vi "display_michelle_PKT_visjitter_stopadded_RandCont_PsuedoCO_TSLogFC1.vi"() -> ()   [LabVIEW 2019]
uses:
  <vilib>/Analysis/Matrix/Datatypes/RealMatrix.ctl
  <vilib>/Utility/file.llb/Write Delimited Spreadsheet (DBL).vi
  <vilib>/Analysis/Matrix/NI_Matrix.lvlib
panel:
  out "savecomplete":bool
  out "lambda":dbl
  out "maxITI":dbl
  out "minITI":dbl
  out "goEXP":dbl
  out "meanITI":dbl
  out "Lag1":dbl
  out "TSLog":dbl[][](array[numeric])
  out "TSLog2":dbl[][](array[numeric])
  out "Initialtime":dbl
  out "Time Stamp":timestamp format="%<%H:%M:%S%4u>T"
  out "TSLog1":dbl[][](array[numeric])
  out "ArrayTemp3":T1
  out "StimID2":dbl
  out "Contrast":dbl
  out "TimeOutCounter":i32
  out "ElapsedTime_M":dbl
  out "Base_Contrast":dbl
  out "CurrentTrial":u32=1
  out "Jitter":dbl
  out "BaseITI":dbl
  out "VisStimDuration":dbl
  in  "Stop":bool
  out "Num trials":u32=204
  out "ISI Time":dbl
  out "Stim TS":dbl
  out "Output":dbl[][](array[numeric])
  out "Output frame":T1
  out "Array temp1":T1
  out "Elapsed Time":dbl
  out "Display":bool=TRUE
  out "Trial":u32=1
  out "reward":dbl[](array[numeric])
  out "stim_id":dbl[](array[numeric])
  out "stim_loaded":dbl
  out "Timings":dbl[](array[numeric])
  out "Stimuli Loaded?":bool
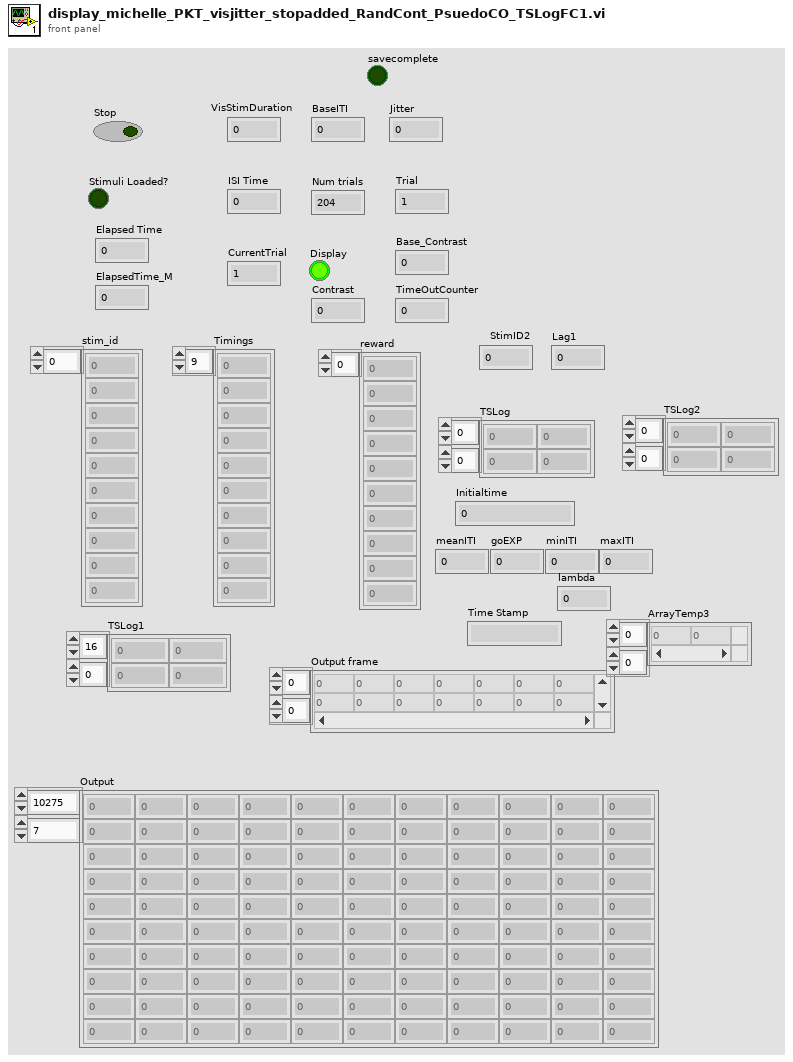
[diagram p1: front panel]
types:
  T1 = typedef "NI_Matrix.lvlib/RealMatrix.ctl" = dbl[][]
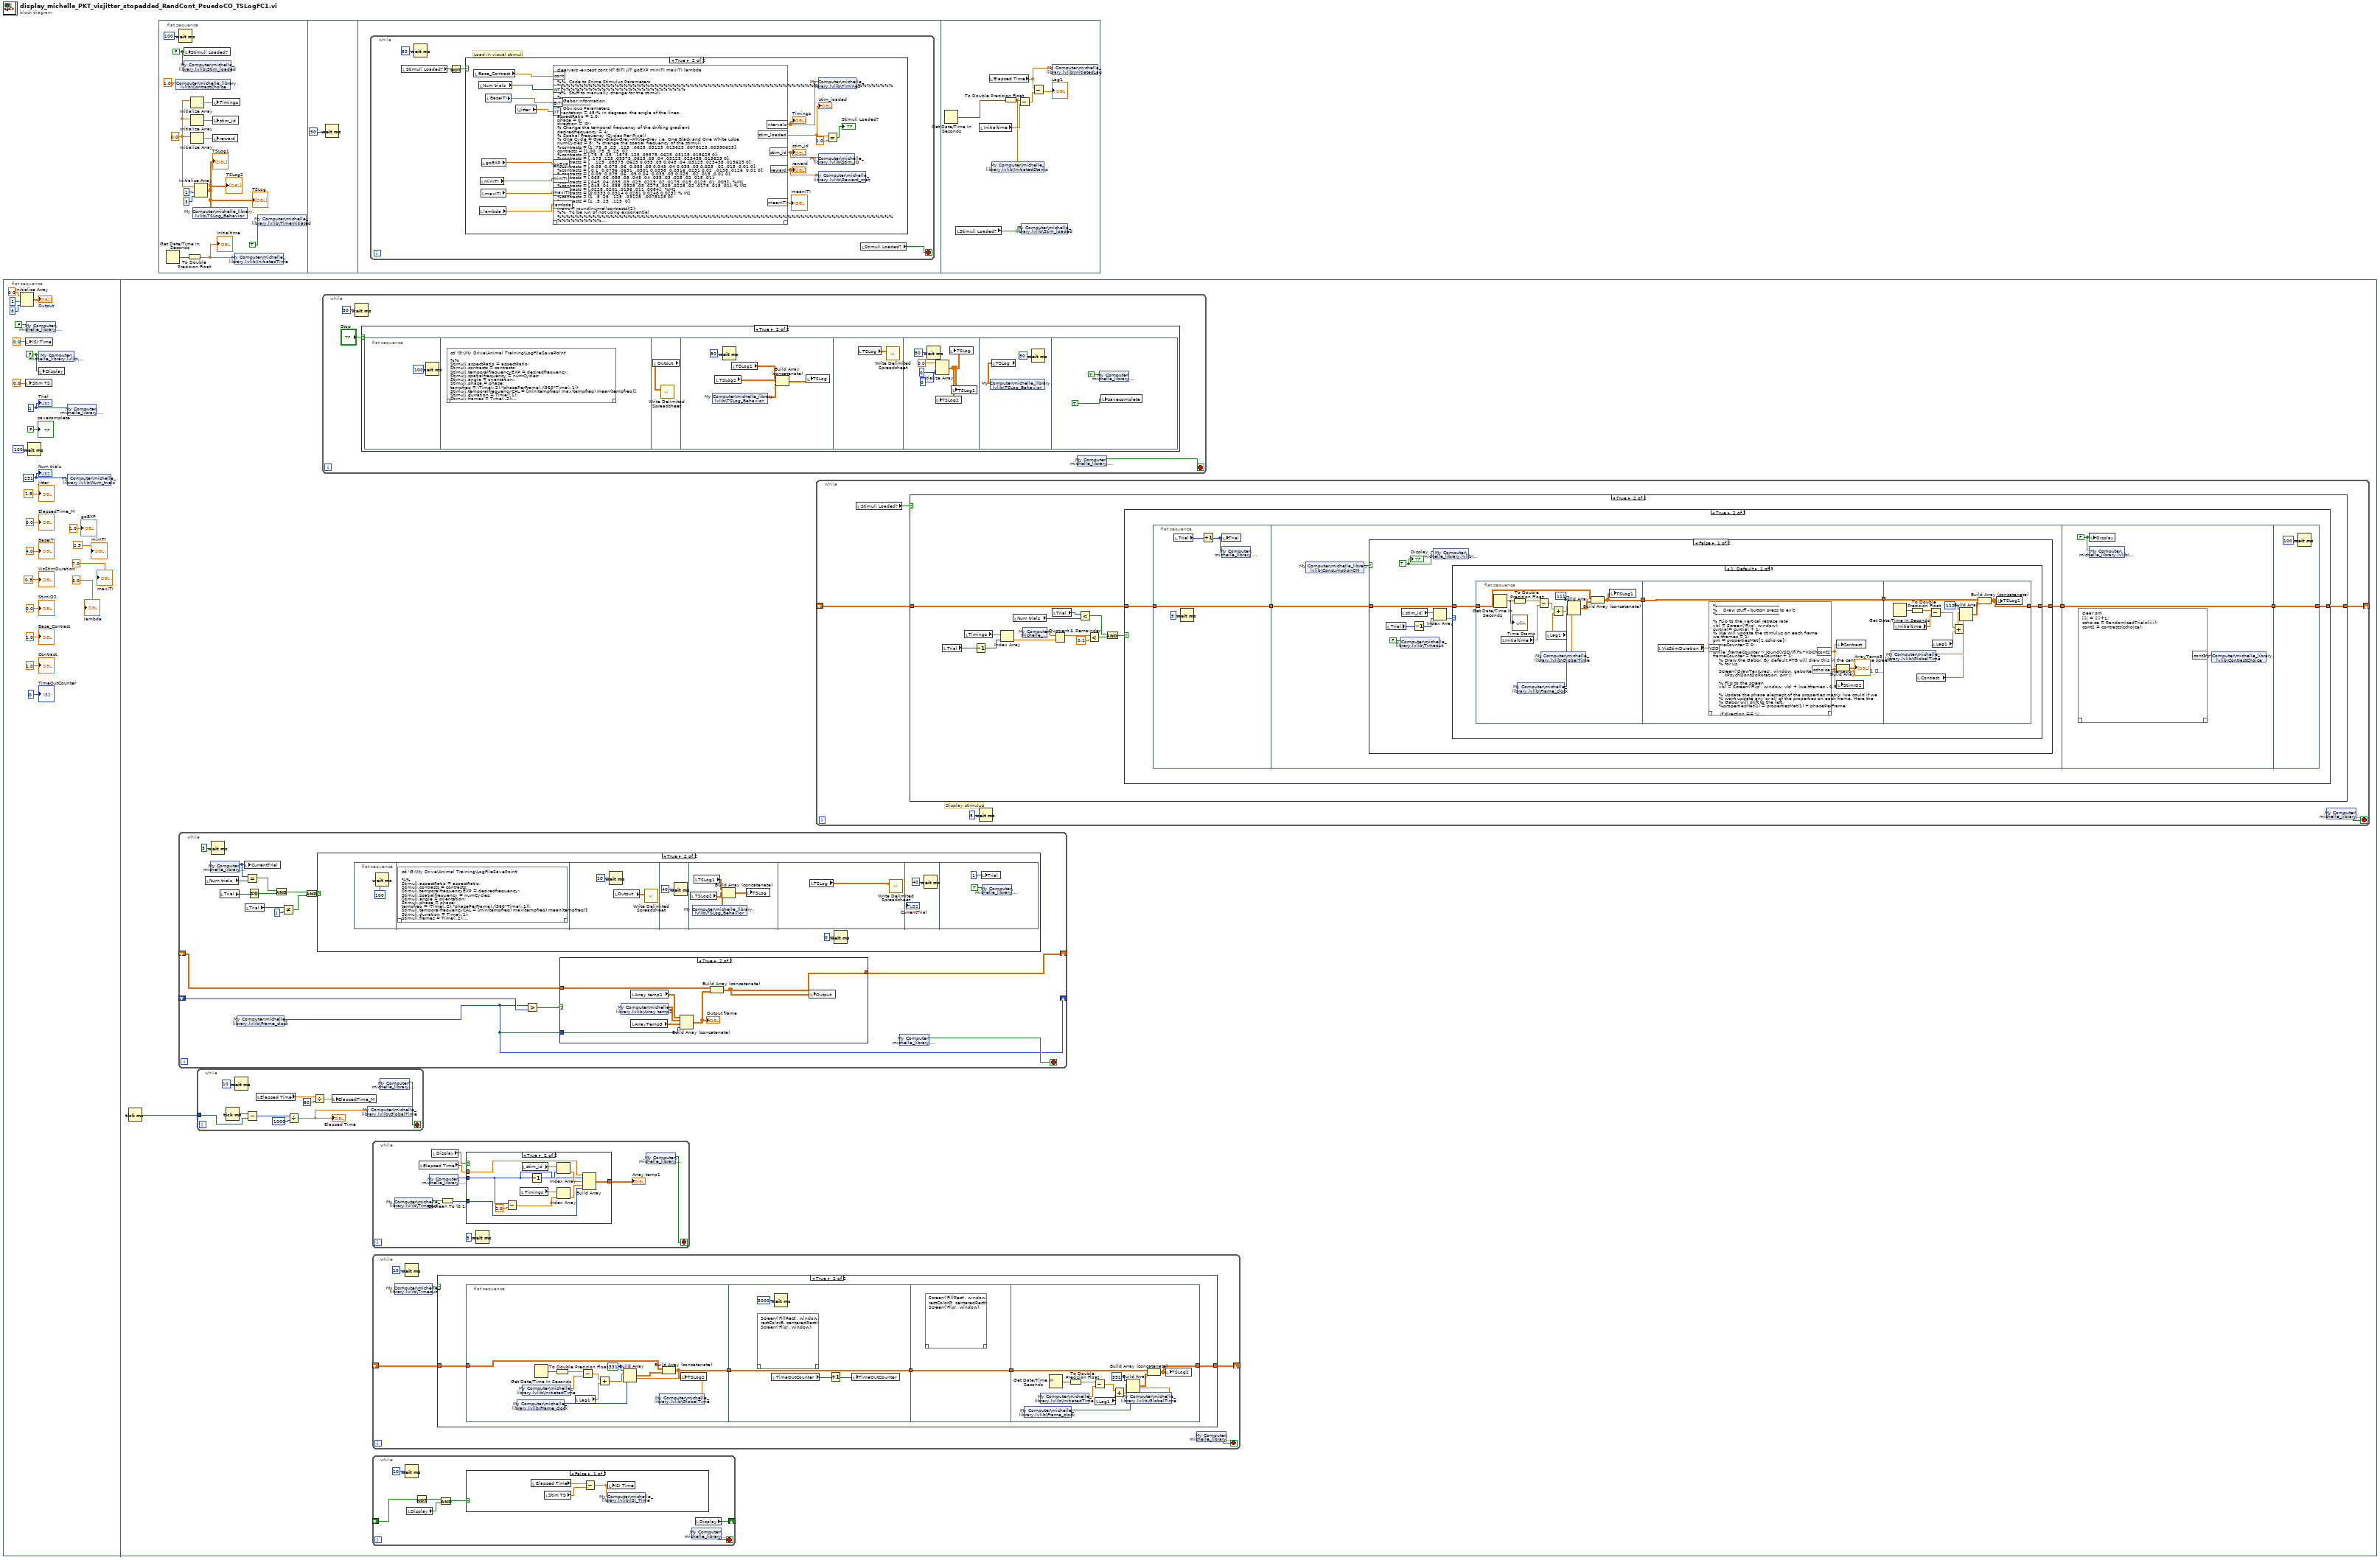
[diagram p0: block diagram]
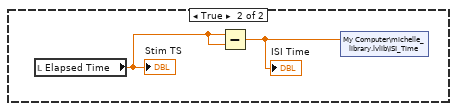
[diagram p5: hidden frame]
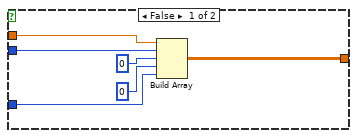
[diagram p6: hidden frame]
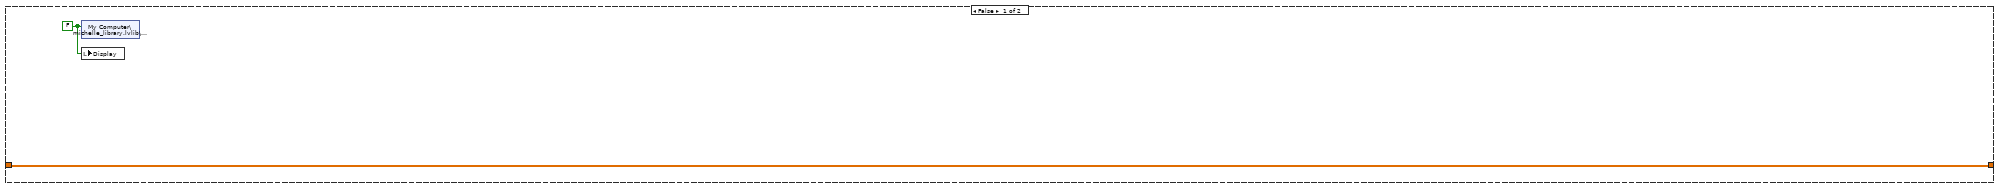
[diagram p10: hidden frame]
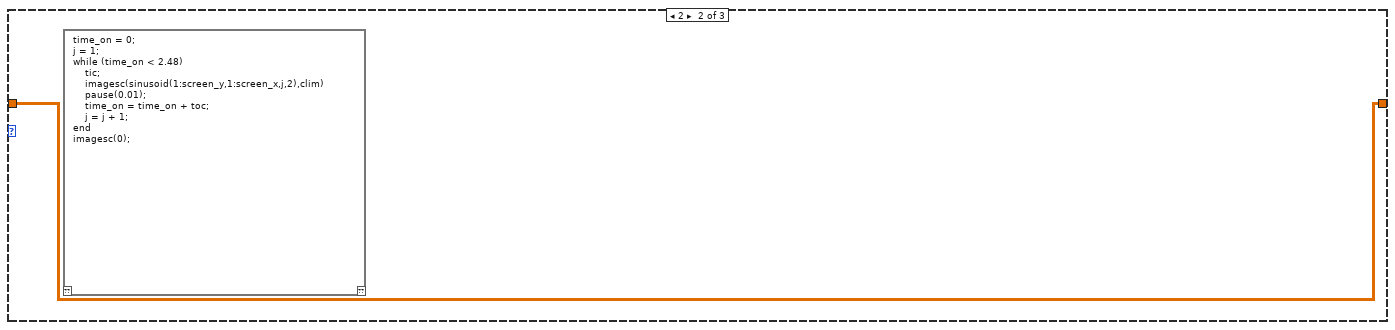
[diagram p11: hidden frame]
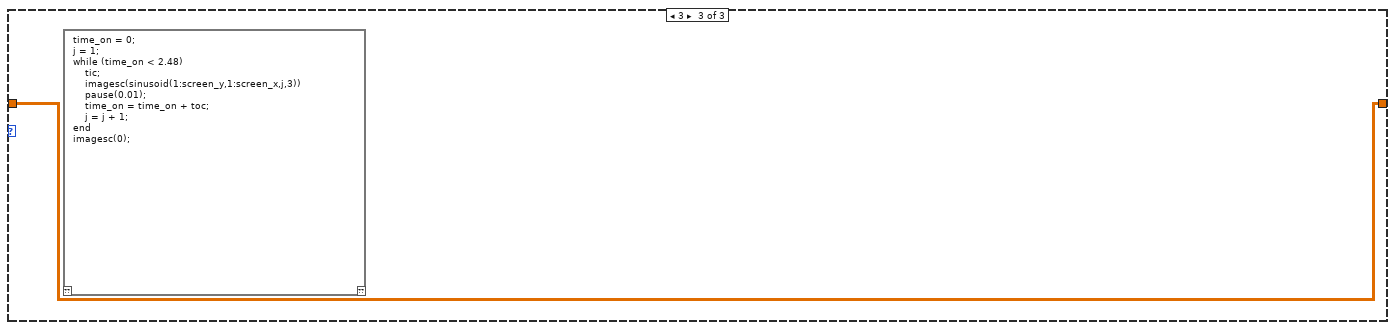
[diagram p12: hidden frame]
diagram:
  n1 = flat-sequence {
    frame #0 {
      w16 = u32 251
      w22 = FALSE ("Display")
      w24 = u32 1 ("Trial")
      n2 = Initialize Array(0.0 ("element"), 1 ("dimension size"), 8 ("dimension size")) -> (→"Output":dbl[][])
      n3 = local write "ISI Time"(0.0 ("ISI Time")) -> ()
      n4 = local write "Stim TS"(0.0 ("Stim TS")) -> ()
      n5 = shared-variable "My Computer\\michelle_library.lvlib\\Stop"(FALSE ("Stop")) -> ()  [unwired: 1 in, 1 out]
      n6 = Wait (ms)(milliseconds to wait=u32 100) -> ()  [unwired: 1 out]
      n7 = shared-variable "My Computer\\michelle_library.lvlib\\Display"(w22) -> ()  [unwired: 1 in, 1 out]
      n8 = local write "Display"(w22) -> ()
      n9 = shared-variable "My Computer\\michelle_library.lvlib\\Trial"(w24) -> ()  [unwired: 1 in, 1 out]
      n10 = shared-variable "My Computer\\michelle_library.lvlib\\Num_trials"(w16) -> ()  [unwired: 1 in, 1 out]
      "Trial" <- w24
      "Num trials" <- w16
      "VisStimDuration" <- 0.5
      "BaseITI" <- 4.0
      "Jitter" <- 1.5
      "Base_Contrast" <- 1.0
      "ElapsedTime_M" <- 0.0
      "TimeOutCounter" <- 0
      "Contrast" <- 1.0
      "StimID2" <- 0.0
      "goEXP" <- 1.0
      "minITI" <- 2.5
      "maxITI" <- 7.0
      "lambda" <- 6.0
      "savecomplete" <- FALSE
    }
    frame #1 {
      n11 = Tick Count (ms)() -> (millisecond timer value=w25:u32)
      n12 = while {
        shift-right: [w136] -> _
        shift-left: _ -> [w137]
        shift-right: [w133] -> _
        shift-left: _ -> [w135]
        stop <- w149 stop-if-true
        n13 = local read "Num trials"() -> (w147:u32)
        n14 = shared-variable "My Computer\\michelle_library.lvlib\\Trial"() -> (w138:u32)  [unwired: 1 in, 1 out]
        n15 = Wait (ms)(milliseconds to wait=u32 3) -> ()  [unwired: 1 out]
        n16 = local read "Trial"() -> (w145:u32)
        n17 = shared-variable "My Computer\\michelle_library.lvlib\\Frame_clock"() -> (w133:u32)  [unwired: 1 in, 1 out]
        n18 = local write "CurrentTrial"(w138) -> ()
        n19 = local read "Trial"() -> (w144:u32)
        n20 = Equal?(x=w138, y=w147) -> (x = y?=w146:bool)
        n21 = Not Equal To 0?(x=w145) -> (x != 0?=w141:bool)
        n22 = And(x=w146, y=w141) -> (x .and. y?=w139:bool)
        n23 = Not Equal?(x=w144, y=1) -> (x != y?=w143:bool)
        n24 = And(x=w139, y=w143) -> (x .and. y?=w140:bool)
        n25 = case shown="True" w140 {
          frame False {
          }
          frame True {
            n26 = flat-sequence {
              frame #0 {
                n27 = Wait (ms)(milliseconds to wait=100) -> ()  [unwired: 1 out]
              }
              frame #1 {
                n28 = script code="cd 'G:\\My Drive\\Animal Training\\LogFileSavePoint'\n\n%%\nStimuli.aspectRatio = aspectRatio;\nStimuli.contrasts = contrasts;\nStimuli.temporalfrequencyEXP = desiredfrequency;\nStimuli.spatialfrequency = numCycles;\nStimuli.angle = orientation;\nStimuli.phase = phase;\ntempfreq = (Time(:,2).*phasePerFrame)./(360*Time(:,1)); \nStimuli.temporalfrequencyCAL = [min(tempfreq) max(tempfreq) mean(tempfreq)];\nStimuli.durration = Time(:,1);\nStimuli.frames = Time(:,2);\nStimuli.contrast = Time(:,3);\nStimuli.intervals = intervals;\nif goEXP == 0\n     int.type = 'jitter';\n     int.baseITI = BITI;\n     int.jitter = JIT;\nelseif goEXP == 1\n     int.type = 'exponential';\n     int.minITI = minITI;\n     int.maxITI = maxITI;\n     int.lambda = lambda;\nend\nStimuli.IntervalData = int;\n\n\nWindow.Xpixels = screenXpixels;\nWindow.Ypixels = screenYpixels;\nWindow.Xcenter = xCenter;\nWindow.Ycenter = yCenter;\nWindow.ifi = ifi;\nWindow.screen = screenNumber;\n\n%%\n[logname] = generatelogname();\n\nsave(logname,'Stimuli','Window');\n\n%%"() -> ()  [unwired: 1 in, 1 out]
              }
              frame #2 {
                n29 = Wait (ms)(milliseconds to wait=u32 10) -> ()  [unwired: 1 out]
                n30 = local read "Output"() -> (w161:dbl[][])
                n31 = call-poly <vilib>:"Write Delimited Spreadsheet.vi"("2D data"=w161) -> ()  [unwired: 13 in, 2 out]
              }
              frame #3 {
                n32 = Wait (ms)(milliseconds to wait=u32 40) -> ()  [unwired: 1 out]
              }
              frame #4 {
                n33 = local read "TSLog2"() -> (w166:dbl[][])
                n34 = shared-variable "My Computer\\michelle_library.lvlib\\TSLog_Behavior"() -> (w164:dbl[][])  [unwired: 1 in, 1 out]
                n35 = local read "TSLog1"() -> (w165:dbl[][])
                n36 = Build Array (concatenate) ("Build Matrix")(w165, w166, w164) -> (w163:T1)
                n37 = local write "TSLog"(w163) -> ()
              }
              frame #5 {
                n38 = local read "TSLog"() -> (w167:dbl[][])
                n39 = call-poly <vilib>:"Write Delimited Spreadsheet.vi"("2D data"=w167) -> ()  [unwired: 13 in, 2 out]
              }
              frame #6 {
                n40 = Wait (ms)(milliseconds to wait=u32 40) -> ()  [unwired: 1 out]
              }
              frame #7 {
                n41 = local write "Trial"(1) -> ()
                n42 = shared-variable "My Computer\\michelle_library.lvlib\\Stop"(TRUE) -> ()  [unwired: 1 in, 1 out]
              }
            }
            n43 = Wait (ms)(milliseconds to wait=0) -> ()  [unwired: 1 out]
          }
        }
        n44 = Greater?(x=w133, y=w135) -> (0:w134:bool)
        n45 = case shown="True" w134 {
          tunnel: w137 -> [w150 w153]
          tunnel: [w150 w152] -> w136
          tunnel: w133 -> [_ w151]
          frame False {
          }
          frame True {
            n46 = shared-variable "My Computer\\michelle_library.lvlib\\Array temp2"() -> (w155:dbl[][])  [unwired: 1 in, 1 out]
            n47 = local read "Array temp1"() -> (w154:T1)
            n48 = local read "ArrayTemp3"() -> (w157:T1)
            n49 = Build Array (concatenate)(w154, w155, w157, w151) -> (w156:T1)
            "Output frame" <- w156
            n50 = Build Array (concatenate) ("Build Matrix")(w153, w156) -> (w152:T1)
            n51 = local write "Output"(w152) -> ()
          }
        }
        n52 = shared-variable "My Computer\\michelle_library.lvlib\\Stop"() -> (w149:bool)  [unwired: 1 in, 1 out]
      }
      n53 = while {
        tunnel: w25 -> [w130]
        stop <- w127 stop-if-true
        n54 = Tick Count (ms)() -> (millisecond timer value=w131:u32)
        n55 = Wait (ms)(milliseconds to wait=u32 10) -> ()  [unwired: 1 out]
        n56 = Subtract(x=w131, y=w130) -> (x-y=w128:u32)
        n57 = local read "Elapsed Time"() -> (w125:dbl)
        n58 = Divide(x=w128, y=u32 1000) -> (x/y=w123:dbl)
        "Elapsed Time" <- w123
        n59 = Divide(x=w125, y=60) -> (x/y=w124:dbl)
        n60 = local write "ElapsedTime_M"(w124) -> ()
        n61 = shared-variable "My Computer\\michelle_library.lvlib\\GlobalTime"(w123) -> ()  [unwired: 1 in, 1 out]
        n62 = shared-variable "My Computer\\michelle_library.lvlib\\Stop"() -> (w127:bool)  [unwired: 1 in, 1 out]
      }
      n63 = while {
        stop <- w26 stop-if-true
        n64 = Wait (ms)(milliseconds to wait=50) -> ()  [unwired: 1 out]
        n65 = case shown="True" "Stop" {
          frame False {
          }
          frame True {
            n66 = flat-sequence {
              frame #0 {
                n67 = Wait (ms)(milliseconds to wait=100) -> ()  [unwired: 1 out]
              }
              frame #1 {
                n68 = script code="cd 'G:\\My Drive\\Animal Training\\LogFileSavePoint'\n\n%%\nStimuli.aspectRatio = aspectRatio;\nStimuli.contrasts = contrasts;\nStimuli.temporalfrequencyEXP = desiredfrequency;\nStimuli.spatialfrequency = numCycles;\nStimuli.angle = orientation;\nStimuli.phase = phase;\ntempfreq = (Time(:,2).*phasePerFrame)./(360*Time(:,1)); \nStimuli.temporalfrequencyCAL = [min(tempfreq) max(tempfreq) mean(tempfreq)];\nStimuli.durration = Time(:,1);\nStimuli.frames = Time(:,2);\nStimuli.contrast = Time(:,3);\nStimuli.intervals = intervals;\nif goEXP == 0\n     int.type = 'jitter';\n     int.baseITI = BITI;\n     int.jitter = JIT;\nelseif goEXP == 1\n     int.type = 'exponential';\n     int.minITI = minITI;\n     int.maxITI = maxITI;\n     int.lambda = lambda;\nend\nStimuli.IntervalData = int;\n\n\nWindow.Xpixels = screenXpixels;\nWindow.Ypixels = screenYpixels;\nWindow.Xcenter = xCenter;\nWindow.Ycenter = yCenter;\nWindow.ifi = ifi;\nWindow.screen = screenNumber;\n\n%%\n[logname] = generatelogname();\n\nsave(logname,'Stimuli','Window');\n\n%%"() -> ()  [unwired: 1 in, 1 out]
              }
              frame #2 {
                n69 = local read "Output"() -> (w30:dbl[][])
                n70 = call-poly <vilib>:"Write Delimited Spreadsheet.vi"("2D data"=w30) -> ()  [unwired: 13 in, 2 out]
              }
              frame #3 {
                n71 = shared-variable "My Computer\\michelle_library.lvlib\\TSLog_Behavior"() -> (w31:dbl[][])  [unwired: 1 in, 1 out]
                n72 = local read "TSLog2"() -> (w34:dbl[][])
                n73 = Wait (ms)(milliseconds to wait=50) -> ()  [unwired: 1 out]
                n74 = local read "TSLog1"() -> (w33:dbl[][])
                n75 = Build Array (concatenate) ("Build Matrix")(w33, w34, w31) -> (w32:T1)
                n76 = local write "TSLog"(w32) -> ()
              }
              frame #4 {
                n77 = local read "TSLog"() -> (w36:dbl[][])
                n78 = call-poly <vilib>:"Write Delimited Spreadsheet.vi"("2D data"=w36) -> ()  [unwired: 13 in, 2 out]
              }
              frame #5 {
                n79 = Wait (ms)(milliseconds to wait=50) -> ()  [unwired: 1 out]
                n80 = Initialize Array(0.0, 0, 0) -> (w38:dbl[][])
                n81 = local write "TSLog2"(w38) -> ()
                n82 = local write "TSLog"(w38) -> ()
                n83 = local write "TSLog1"(w38) -> ()
              }
              frame #6 {
                n84 = local read "TSLog"() -> (w43:dbl[][])
                n85 = shared-variable "My Computer\\michelle_library.lvlib\\TSLog_Behavior"(w43) -> ()  [unwired: 1 in, 1 out]
                n86 = Wait (ms)(milliseconds to wait=50) -> ()  [unwired: 1 out]
              }
              frame #7 {
                n87 = shared-variable "My Computer\\michelle_library.lvlib\\Stop"(TRUE) -> ()  [unwired: 1 in, 1 out]
                n88 = local write "savecomplete"(TRUE) -> ()
              }
            }
          }
        }
        n89 = shared-variable "My Computer\\michelle_library.lvlib\\Stop"() -> (w26:bool)  [unwired: 1 in, 1 out]
      }
      n90 = while {
        stop <- w100 stop-if-true
        n91 = shared-variable "My Computer\\michelle_library.lvlib\\Timeout"() -> (w98:bool)  [unwired: 1 in, 1 out]
        n92 = local read "Elapsed Time"() -> (w104:dbl)
        n93 = shared-variable "My Computer\\michelle_library.lvlib\\Trial"() -> (w102:u32)  [unwired: 1 in, 1 out]
        n94 = local read "Display"() -> (w101:bool)
        n95 = Boolean To (0,1)(Boolean=w98) -> (0, 1=w99:i16)
        n96 = case shown="True" w101 {
          tunnel: w102 -> [w110 w113]
          tunnel: w104 -> [w111 w120]
          tunnel: [w109 w121] -> w103
          tunnel: w99 -> [w106 w115]
          frame False {
            n97 = Build Array(w111, w110, u32 0 ("milliseconds to wait"), 0, w106) -> (w109:T1)
          }
          frame True {
            n98 = Subtract(x=w113, y=2.0) -> (x-y=w112:dbl)
            n99 = local read "Timings"() -> (w118:dbl[])
            n100 = local read "stim_id"() -> (w122:dbl[])
            n101 = Decrement(x=w113) -> (x-1=w117:u32)
            n102 = Index Array(array=w122, index=w117) -> (element=w119:dbl)
            n103 = Index Array(array=w118, index=w112) -> (element=w116:dbl)
            n104 = Build Array(w120, w113, w119, w116, w115) -> (w121:T1)
          }
        }
        "Array temp1" <- w103
        n105 = Wait (ms)(milliseconds to wait=u32 5) -> ()  [unwired: 1 out]
        n106 = shared-variable "My Computer\\michelle_library.lvlib\\Stop"() -> (w100:bool)  [unwired: 1 in, 1 out]
      }
      n107 = while {
        shift-right: [w46] -> _
        shift-left: _ -> [w47]
        stop <- w50 stop-if-true
        n108 = shared-variable "My Computer\\michelle_library.lvlib\\Timeout"() -> (w48:bool)  [unwired: 1 in, 1 out]
        n109 = Wait (ms)(milliseconds to wait=u32 10) -> ()  [unwired: 1 out]
        n110 = case shown="True" w48 {
          tunnel: w47 -> [w51 w56]
          tunnel: [w51 w55] -> w46
          frame False {
          }
          frame True {
            n111 = flat-sequence {
              tunnel: w56 -> [w63]
              tunnel: [w62] -> w53
              tunnel: [w69] -> w54
              tunnel: w53 -> [w69]
              tunnel: w54 -> [w73]
              tunnel: [w73] -> w52
              tunnel: [w79] -> w55
              tunnel: w52 -> [w80]
              frame #0 {
                n112 = shared-variable "My Computer\\michelle_library.lvlib\\Frame_clock"() -> (w57:u32)  [unwired: 1 in, 1 out]
                n113 = shared-variable "My Computer\\michelle_library.lvlib\\InitiatedTime"() -> (w66:dbl)  [unwired: 1 in, 1 out]
                n114 = Get Date/Time In Seconds() -> (seconds since 1Jan1904=w68:timestamp)
                n115 = To Double Precision Float(number=w68) -> (double precision float=w67:dbl)
                n116 = local read "Lag1"() -> (w59:dbl)
                n117 = Subtract(x=w67, y=w66) -> (x-y=w60:dbl)
                n118 = Add(x=w60, y=w59) -> (x+y=w61:dbl)
                n119 = shared-variable "My Computer\\michelle_library.lvlib\\GlobalTime"() -> (w58:dbl)  [unwired: 1 in, 1 out]
                n120 = Build Array(331, w61, w58, w57) -> (w65:T1)
                n121 = Build Array (concatenate) ("Build Matrix")(w63, w65) -> (w62:T1)
                n122 = local write "TSLog2"(w62) -> ()
              }
              frame #1 {
                n123 = script code="Screen('FillRect', window, rectColorB, centeredRect);\nScreen('Flip', window);"() -> ()  [unwired: 1 in, 1 out]
                n124 = local read "TimeOutCounter"() -> (w71:i32)
                n125 = Wait (ms)(milliseconds to wait=u32 3000) -> ()  [unwired: 1 out]
                n126 = Increment(x=w71) -> (x+1=w70:i32)
                n127 = local write "TimeOutCounter"(w70) -> ()
              }
              frame #2 {
                n128 = script code="Screen('FillRect', window, rectColorG, centeredRect);\nScreen('Flip', window);"() -> ()  [unwired: 1 in, 1 out]
              }
              frame #3 {
                n129 = shared-variable "My Computer\\michelle_library.lvlib\\Frame_clock"() -> (w74:u32)  [unwired: 1 in, 1 out]
                n130 = shared-variable "My Computer\\michelle_library.lvlib\\InitiatedTime"() -> (w85:dbl)  [unwired: 1 in, 1 out]
                n131 = Get Date/Time In Seconds() -> (seconds since 1Jan1904=w83:timestamp)
                n132 = To Double Precision Float(number=w83) -> (double precision float=w84:dbl)
                n133 = Subtract(x=w84, y=w85) -> (x-y=w77:dbl)
                n134 = local read "Lag1"() -> (w76:dbl)
                n135 = Add(x=w77, y=w76) -> (x+y=w78:dbl)
                n136 = shared-variable "My Computer\\michelle_library.lvlib\\GlobalTime"() -> (w75:dbl)  [unwired: 1 in, 1 out]
                n137 = Build Array(332, w78, w75, w74) -> (w81:T1)
                n138 = Build Array (concatenate) ("Build Matrix")(w80, w81) -> (w79:T1)
                n139 = local write "TSLog2"(w79) -> ()
              }
            }
          }
        }
        n140 = shared-variable "My Computer\\michelle_library.lvlib\\Stop"() -> (w50:bool)  [unwired: 1 in, 1 out]
      }
      n141 = while {
        shift-right: [w90] -> _
        shift-left: _ -> [w89]
        stop <- w92 stop-if-true
        n142 = Wait (ms)(milliseconds to wait=u32 10) -> ()  [unwired: 1 out]
        n143 = local read "Display"() -> (w87:bool)
        n144 = Not(x=w89) -> (.not. x?=w88:bool)
        n145 = And(x=w88, y=w87) -> (x .and. y?=w86:bool)
        n146 = case shown="False" w86 {
          frame False {
            n147 = local read "Elapsed Time"() -> (w93:dbl)
            n148 = local read "Stim TS"() -> (w95:dbl)
            n149 = Subtract(x=w93, y=w95) -> (x-y=w94:dbl)
            n150 = local write "ISI Time"(w94) -> ()
            n151 = shared-variable "My Computer\\michelle_library.lvlib\\ISI_Time"(w94) -> ()  [unwired: 1 in, 1 out]
          }
          frame True {
            n152 = local read "Elapsed Time"() -> (w96:dbl)
            "Stim TS" <- w96
            n153 = Subtract(x=w96, y=w96) -> (x-y=w97:dbl)
            "ISI Time" <- w97
            n154 = shared-variable "My Computer\\michelle_library.lvlib\\ISI_Time"(w97) -> ()  [unwired: 1 in, 1 out]
          }
        }
        n155 = shared-variable "My Computer\\michelle_library.lvlib\\Stop"() -> (w92:bool)  [unwired: 1 in, 1 out]
        n156 = local read "Display"() -> (w90:bool)
      }
      n157 = while {
        shift-right: [w171] -> _
        shift-left: _ -> [w172]
        stop <- w174 stop-if-true
        # "Display stimulus"
        n158 = local read "Stimuli Loaded?"() -> (w173:bool)
        n159 = case shown="True" w173 {
          tunnel: w172 -> [w176 w178]
          tunnel: [w176 w177] -> w171
          frame False {
          }
          frame True {
            n160 = local read "Trial"() -> (w179:u32)
            n161 = local read "Timings"() -> (w188:dbl[])
            n162 = Decrement(x=w179) -> (x-1=w180:u32)
            n163 = Index Array(array=w188, index=w180) -> (element=w187:dbl)
            n164 = local read "Num trials"() -> (w183:u32)
            n165 = shared-variable "My Computer\\michelle_library.lvlib\\ISI"() -> (w182:dbl)  [unwired: 1 in, 1 out]
            n166 = local read "Trial"() -> (w186:u32)
            n167 = Quotient & Remainder(x=w182, y=w187) -> (x-y*floor(x/y)=w190:dbl)  [unwired: 1 out]
            n168 = Less?(x=w186, y=w183) -> (x < y?=w185:bool)
            n169 = Less?(x=w190, y=0.1) -> (x < y?=w184:bool)
            n170 = And(x=w185, y=w184) -> (x .and. y?=w181:bool)
            n171 = case shown="True" w181 {
              tunnel: w178 -> [w191 w196]
              tunnel: [w191 w195] -> w177
              frame False {
                w192 = FALSE ("Display")
                n172 = shared-variable "My Computer\\michelle_library.lvlib\\Display"(w192) -> ()  [unwired: 1 in, 1 out]
                n173 = local write "Display"(w192) -> ()
              }
              frame True {
                n174 = flat-sequence {
                  tunnel: [w198] -> w197
                  tunnel: w196 -> [w198]
                  tunnel: w197 -> [w203]
                  tunnel: [w202] -> w193
                  tunnel: [w249] -> w194
                  tunnel: w193 -> [w249]
                  tunnel: [w252] -> w195
                  tunnel: w194 -> [w252]
                  frame #0 {
                    n175 = local read "Trial"() -> (w201:u32)
                    n176 = Wait (ms)(milliseconds to wait=u32 5) -> ()  [unwired: 1 out]
                    n177 = Increment(x=w201) -> (x+1=w200:u32)
                    n178 = local write "Trial"(w200) -> ()
                    n179 = shared-variable "My Computer\\michelle_library.lvlib\\Trial"(w200) -> ()  [unwired: 1 in, 1 out]
                  }
                  frame #1 {
                    n180 = shared-variable "My Computer\\michelle_library.lvlib\\ConsumptionON"() -> (w204:bool)  [unwired: 1 in, 1 out]
                    n181 = case shown="False" w204 {
                      tunnel: w203 -> [w206 w248]
                      tunnel: [w205 w248] -> w202
                      frame False {
                        w207 = TRUE ("Boolean")
                        n182 = local read "Trial"() -> (w210:u32)
                        n183 = shared-variable "My Computer\\michelle_library.lvlib\\Timeout"(FALSE) -> ()  [unwired: 1 in, 1 out]
                        n184 = local read "stim_id"() -> (w212:dbl[])
                        n185 = Decrement(x=w210) -> (x-1=w209:u32)
                        n186 = shared-variable "My Computer\\michelle_library.lvlib\\Display"(w207) -> ()  [unwired: 1 in, 1 out]
                        n187 = Index Array(array=w212, index=w209) -> (element=w211:dbl)
                        n188 = case shown="1, Default" w211 {
                          tunnel: w206 -> [w216 w246 w247]
                          tunnel: [w215 w246 w247] -> w205
                          frame 1, Default {
                            n189 = flat-sequence {
                              tunnel: w216 -> [w227]
                              tunnel: [w226] -> w214
                              tunnel: w214 -> [w229]
                              tunnel: [w229] -> w213
                              tunnel: [w244] -> w215
                              tunnel: w213 -> [w243]
                              frame #0 {
                                n190 = Get Date/Time In Seconds() -> (seconds since 1Jan1904=w224:timestamp)
                                "Time Stamp" <- w224
                                n191 = local read "Initialtime"() -> (w222:dbl)
                                n192 = To Double Precision Float(number=w224) -> (double precision float=w223:dbl)
                                n193 = shared-variable "My Computer\\michelle_library.lvlib\\Frame_clock"() -> (w217:u32)  [unwired: 1 in, 1 out]
                                n194 = Subtract(x=w223, y=w222) -> (x-y=w220:dbl)
                                n195 = shared-variable "My Computer\\michelle_library.lvlib\\GlobalTime"() -> (w218:dbl)  [unwired: 1 in, 1 out]
                                n196 = local read "Lag1"() -> (w221:dbl)
                                n197 = Add(x=w220, y=w221) -> (x+y=w219:dbl)
                                n198 = Build Array(111, w219, w218, w217) -> (w225:T1)
                                n199 = Build Array (concatenate) ("Build Matrix")(w227, w225) -> (w226:T1)
                                n200 = local write "TSLog1"(w226) -> ()
                              }
                              frame #1 {
                                n201 = local read "VisStimDuration"() -> (w231:dbl)
                                n202 = script code="%------------------------------------------\n%    Draw stuff - button press to exit\n%------------------------------------------\n\n% FLip to the vertical retrace rate\nvbl = Screen('Flip', window);\ncurtrial= curtrial + 1;\n% We will update the stimulus on each frame\nwaitframes = 1;\npm = propertiesMat{1,cchoice};\nframeCounter = 0;\ntic\nwhile  frameCounter < round(VSD/ifi)%~KbCheck\nframeCounter = frameCounter + 1;\n    % Draw the Gabor. By default PTB will draw this in the center of the screen\n    % for us.\n   \n    Screen('DrawTextures', window, gabortex, [], [], orientation, [], [], [], [],...\n        kPsychDontDoRotation, pm');\n\n    % Flip to the screen\n    vbl = Screen('Flip', window, vbl + (waitframes - 0.5) * ifi);\n\n    % Update the phase element of the properties matrix (we could if we\n    % want update any or all of the properties on each frame. Here the\n    % Gabor will drift to the left.\n    %propertiesMat(1) = propertiesMat(1) + phasePerFrame;\n \n     if direction == 'L'\n          pm(1) = pm(1) + phasePerFrame;\n     elseif direction =='R'\n          pm(1) = pm(1) - phasePerFrame;\n     end\n\nend\nTime(curtrial,1) = toc;\nTime(curtrial,2) = frameCounter;\nTime(curtrial,3) = pm(4);\nvbl = Screen('Flip', window);"("VSD"=w231) -> ("cont2"=w233:dbl, "cchoice"=w232:dbl)  [unwired: 1 in, 1 out]
                                n203 = local write "Contrast"(w233) -> ()
                                n204 = Build Array(w233, w232) -> (→"ArrayTemp3":T1)
                                n205 = local write "StimID2"(w232) -> ()
                              }
                              frame #2 {
                                n206 = shared-variable "My Computer\\michelle_library.lvlib\\GlobalTime"() -> (w235:dbl)  [unwired: 1 in, 1 out]
                                n207 = Get Date/Time In Seconds() -> (seconds since 1Jan1904=w241:timestamp)
                                n208 = local read "Initialtime"() -> (w240:dbl)
                                n209 = To Double Precision Float(number=w241) -> (double precision float=w239:dbl)
                                n210 = local read "Contrast"() -> (w234:dbl)
                                n211 = Subtract(x=w239, y=w240) -> (x-y=w238:dbl)
                                n212 = local read "Lag1"() -> (w236:dbl)
                                n213 = Add(x=w238, y=w236) -> (x+y=w237:dbl)
                                n214 = Build Array(112, w237, w235, w234) -> (w245:T1)
                                n215 = Build Array (concatenate) ("Build Matrix")(w243, w245) -> (w244:T1)
                                n216 = local write "TSLog1"(w244) -> ()
                              }
                            }
                          }
                          frame 2 {
                            n217 = script code="time_on = 0;\nj = 1;\nwhile (time_on < 2.48)\n    tic;\n    imagesc(sinusoid(1:screen_y,1:screen_x,j,2),clim)\n    pause(0.01);\n    time_on = time_on + toc;\n    j = j + 1;\nend\nimagesc(0);"() -> ()  [unwired: 1 in, 1 out]
                          }
                          frame 3 {
                            n218 = script code="time_on = 0;\nj = 1;\nwhile (time_on < 2.48)\n    tic;\n    imagesc(sinusoid(1:screen_y,1:screen_x,j,3))\n    pause(0.01);\n    time_on = time_on + toc;\n    j = j + 1;\nend\nimagesc(0);"() -> ()  [unwired: 1 in, 1 out]
                          }
                        }
                        "Display" <- w207
                      }
                      frame True {
                      }
                    }
                  }
                  frame #2 {
                    w251 = FALSE ("Display")
                    n219 = script code="clear pm\niiii = iiii+1;\ncchoice = RandomizedTrials(iiii);\ncont2 = contrasts(cchoice);"() -> ("cont2"=w250:dbl)  [unwired: 1 in, 1 out]
                    n220 = local write "Display"(w251) -> ()
                    n221 = shared-variable "My Computer\\michelle_library.lvlib\\Display"(w251) -> ()  [unwired: 1 in, 1 out]
                    n222 = shared-variable "My Computer\\michelle_library.lvlib\\ContrastChoice"(w250) -> ()  [unwired: 1 in, 1 out]
                  }
                  frame #3 {
                    n223 = Wait (ms)(milliseconds to wait=u32 100) -> ()  [unwired: 1 out]
                  }
                }
              }
            }
          }
        }
        n224 = Wait (ms)(milliseconds to wait=u32 5) -> ()  [unwired: 1 out]
        n225 = shared-variable "My Computer\\michelle_library.lvlib\\Stop"() -> (w174:bool)  [unwired: 1 in, 1 out]
      }
    }
  }
  n226 = flat-sequence {
    frame #0 {
      w260 = 0.0 ("element")
      w262 = FALSE ("Stimuli Loaded?")
      n227 = Get Date/Time In Seconds() -> (seconds since 1Jan1904=w257:timestamp)
      n228 = shared-variable "My Computer\\michelle_library.lvlib\\ContrastChoice"(1.0) -> ()  [unwired: 1 in, 1 out]
      n229 = Wait (ms)(milliseconds to wait=u32 100) -> ()  [unwired: 1 out]
      n230 = local write "Stimuli Loaded?"(w262) -> ()
      n231 = shared-variable "My Computer\\michelle_library.lvlib\\Stim_loaded"(w262) -> ()  [unwired: 1 in, 1 out]
      n232 = To Double Precision Float(number=w257) -> (double precision float=w256:dbl)
      "Initialtime" <- w256
      n233 = Initialize Array(w260) -> (w265:dbl[])  [unwired: 1 in]
      n234 = Initialize Array(w260) -> (w264:dbl[])  [unwired: 1 in]
      n235 = Initialize Array(w260) -> (w263:dbl[])  [unwired: 1 in]
      n236 = Initialize Array(w260, 1, 3) -> (w254:dbl[][])
      "TSLog1" <- w254
      "TSLog2" <- w254
      "TSLog" <- w254
      n237 = shared-variable "My Computer\\michelle_library.lvlib\\TSLog_Behavior"(w254) -> ()  [unwired: 1 in, 1 out]
      n238 = local write "Timings"(w265) -> ()
      n239 = local write "stim_id"(w264) -> ()
      n240 = local write "reward"(w263) -> ()
      n241 = shared-variable "My Computer\\michelle_library.lvlib\\InitiatedTime"(w256) -> ()  [unwired: 1 in, 1 out]
      n242 = shared-variable "My Computer\\michelle_library.lvlib\\TimeInitiated"(TRUE) -> ()  [unwired: 1 in, 1 out]
    }
    frame #1 {
      n243 = Wait (ms)(milliseconds to wait=u32 50) -> ()  [unwired: 1 out]
    }
    frame #2 {
      n244 = while {
        stop <- w268 stop-if-true
        # "Load in visual stimuli"
        n245 = local read "Stimuli Loaded?"() -> (w270:bool)
        n246 = Wait (ms)(milliseconds to wait=u32 50) -> ()  [unwired: 1 out]
        n247 = Not(x=w270) -> (.not. x?=w269:bool)
        n248 = case shown="True" w269 {
          frame False {
          }
          frame True {
            n249 = local read "Base_Contrast"() -> (w278:dbl)
            n250 = local read "Num trials"() -> (w281:u32)
            n251 = local read "lambda"() -> (w272:dbl)
            n252 = local read "minITI"() -> (w274:dbl)
            n253 = local read "maxITI"() -> (w273:dbl)
            n254 = local read "goEXP"() -> (w275:dbl)
            n255 = local read "BaseITI"() -> (w280:dbl)
            n256 = local read "Jitter"() -> (w279:dbl)
            n257 = script code="clearvars -except cont NT BITI JIT goEXP minITI maxITI lambda\n\n\n%%  Code to Prime Stimulus Parameters\n%%%%%%%%%%%%%%%%%%%%%%%%%%%%%%%%%%%%%%%%%%%%%%%%%%%%%%%%%%%%%%%%%%%%%%%%%%%%%%%%%%%%%%%%%%%%%%%%%%%%%%%%%\n%%  Stuff to manually change for the stimuli\n%--------------------\n% Gabor information\n%--------------------\n% Obvious Parameters\norientation = 45;% in degrees, the angle of the lines.\naspectRatio = 1.0;\nphase = 0;\ndirection = 'R';\n% Change the temporal frequency of the drifting gradient\ndesiredfrequency = 4;\n% Spatial Frequency (Cycles Per Pixel)\n% One Cycle = Grey-Black-Grey-White-Grey i.e. One Black and One White Lobe\nnumCycles = 8;  % change the spatial frequency of the stimuli\n%contrasts = [1 .75 .5 .25  .125  .0625 .03125 .015625 .0078125 .00390625];\ncontrasts = [1.00 .75 .5 .25  0];\n%contrasts = [.75 .5 .25  .1875 .125 .09375 .0625 .03125 .015625 0];\n%contrasts = [ .175 .125 .09375 .0625 .05 .04 .03125 .023438 .015625 0];\n%contrasts = [   .125  .09375 .0625 0.055 .05 0.045 .04 .03125 .023438 .015625 0];\n%contrasts = [ 0.09  0.075 .06  0.055 .05 0.045 .04 0.035 .03 0.025  .02 .015  0.01 0];\n%contrasts = [ 0.1  0.0796 .0631  .0501 0.0398  0.0316 .0251 0.02  .0158 .0126  0.01 0];\n%contrasts = [ 0.09  0.075 .06  .05 0.04  0.035 .03 0.025  .02 .015  0.01 0];\n%contrasts = [.065 .06 .055 .05 .045 .04 .035 .03 .025 .02 .015 .01];\n%contrasts = [.045 .04 .035 .03 .025 .0225 .02 .0175 .015 .0125 .01 .005];  %M1\n%contrasts = [.045 .04 .035 .0325 .03 .0275 .025 .0225 .02 .0175 .015 .01]; % M2\n%contrasts = [.0228 .0201 .0156 .011 .0084];  %M1\n%contrasts = [0.0333 0.0314 0.0281 0.0248 0.023]; % M2\n%contrasts = [1  .5 .25  .125  .03125  .0078125 0];\n%contrasts = [1  .5 .25  .125  0];\ngo = 1;\nmaxc = round(numel(contrasts)/2);\n%%  To be run of not using exponential\n%%%%%%%%%%%%%%%%%%%%%%%%%%%%%%%%%%%%%%%%%%%%%%%%%%%%%%%%%%%%%%%%%%%%%%%%%%%%%%%%%%%%%%\n% This code will randomize the order of contrasts being presented\n[RandomizedTrials]=RandomizeTrials_Psuedo_function(contrasts,NT,'n');\n\n% This code will generate inter trial intervals with either random jitter\n% or based on an exponential distribution\nif goEXP < 1\n     jit = JIT;\n     jitter = rand(1,NT);\n     jitter = 2*jit*(jitter- .5);\n     ITIbase = BITI;\n     intervals = [ones(1,NT)*ITIbase];\n     intervals = intervals + jitter;\nelseif goEXP > 0\n     intervals = exponentialITI(1/lambda, minITI, maxITI, NT);\nend\n\n%%  Prep the stimulus presentation software\n%%%%%%%%%%%%%%%%%%%%%%%%%%%%%%%%%%%%%%%%%%%%%%%%%%%%%%%%%%%%%%%%%%%%%%%%%%%\n%Screen('Preference', 'SkipSyncTests', 1);\nsca;\nclose all;\n% Setup PTB with some default values\nPsychDefaultSetup(2);\n% Set the screen number to the external secondary monitor if there is one connected\nscreenNumber = max(Screen('Screens'));\n\n% Define black, white and grey\nwhite = WhiteIndex(screenNumber);\nblack = BlackIndex(screenNumber);\ngrey = white / 2;\n\n% Open the screen & define it's dimensions\n[window, windowRect] = PsychImaging('OpenWindow', screenNumber, grey,...\n    [], 32, 2, [], [], kPsychNeedRetinaResolution);\n[screenXpixels, screenYpixels] = Screen('WindowSize', window);\n[xCenter, yCenter] = RectCenter(windowRect);\n\n% Get the vertical refresh rate of the monitor\nifi = Screen('GetFlipInterval', window);\n\n% Set maximum priority level\ntopPriorityLevel = MaxPriority(window);\nPriority(topPriorityLevel);\n\n\n% Build a procedural gabor texture (Note: to get a \"standard\" Gabor patch\n% we set a grey background offset, disable normalisation, and set a\n% pre-contrast multiplier of 0.5).\n% Dimension of the region where will draw the Gabor in pixels\ngaborDimPix = windowRect(3);\n% Sigma of Gaussian  (how much to fade around the edges)\nsigma = gaborDimPix / 0;  % change the 0 value to alter the fading\nphasePerFrame = desiredfrequency*360*ifi;\nfreq = numCycles / gaborDimPix;\n\nbackgroundOffset = [0.5 0.5 0.5 0.0];\ndisableNorm = 1;\npreContrastMultiplier = 0.5;\ngabortex = CreateProceduralGabor(window, gaborDimPix, gaborDimPix, [],...\n    backgroundOffset, disableNorm, preContrastMultiplier);\n\n% Randomise the phase of the Gabors and make a properties matrix.\nfor N = 1:numel(contrasts)\npropertiesMat{1,N} = [phase, freq, sigma, contrasts(N), aspectRatio, 0, 0, 0];\nend\n\niiii = 1;\ncchoice = RandomizedTrials(iiii);\ncont2 = contrasts(cchoice);\npm = propertiesMat{1,1};\ncurtrial = 0;\n\n%%  Build up the rectangles for the pause and hold screen\nbaseRect = [0 0 screenXpixels screenYpixels];\ncenteredRect = CenterRectOnPointd(baseRect, xCenter, yCenter);\nrectColorB = [0 0 0];\nrectColorG = [128 128 128]/255;\n\n%%  Finalize the trial data and orders\nstim_id = [ones(1,NT)*1];\nreward = [ones(1,NT)*1];\nmeanITI = nanmean(intervals);\nrand_idx1 = randperm(NT);\nrand_idx2 = randperm(NT);\nintervals = intervals(rand_idx2);\nstim_id = stim_id(rand_idx2);\nreward = reward(rand_idx2);\n%%  All Done!\n%  indicate that the necessary preloading of data has been completed.\nstim_loaded = 1;" ("Script Node")("NT"=w281, "BITI"=w280, "JIT"=w279, "cont"=w278, "goEXP"=w275, "minITI"=w274, "maxITI"=w273, "lambda"=w272) -> ("stim_loaded"=w286:dbl, "intervals"=w282:dbl[], "stim_id"=w283:dbl[], "reward"=w284:dbl[], "meanITI"=→"meanITI":dbl)  [unwired: 1 in, 1 out]
            "stim_loaded" <- w286
            "Timings" <- w282
            "stim_id" <- w283
            "reward" <- w284
            n258 = shared-variable "My Computer\\michelle_library.lvlib\\Timings"(w282) -> ()  [unwired: 1 in, 1 out]
            n259 = shared-variable "My Computer\\michelle_library.lvlib\\Stim_ID"(w283) -> ()  [unwired: 1 in, 1 out]
            n260 = shared-variable "My Computer\\michelle_library.lvlib\\Reward_mat"(w284) -> ()  [unwired: 1 in, 1 out]
            n261 = Equal?(x=w286, y=1.0) -> (x = y?=→"Stimuli Loaded?":bool)
          }
        }
        n262 = local read "Stimuli Loaded?"() -> (w268:bool)
      }
    }
    frame #3 {
      n263 = Get Date/Time In Seconds() -> (seconds since 1Jan1904=w293:timestamp)
      n264 = local read "Stimuli Loaded?"() -> (w288:bool)
      n265 = local read "Initialtime"() -> (w292:dbl)
      n266 = local read "Elapsed Time"() -> (w287:dbl)
      n267 = To Double Precision Float(number=w293) -> (double precision float=w290:dbl)
      n268 = shared-variable "My Computer\\michelle_library.lvlib\\InitiatedStamp"(w290) -> ()  [unwired: 1 in, 1 out]
      n269 = Subtract(x=w290, y=w292) -> (x-y=w291:dbl)
      n270 = shared-variable "My Computer\\michelle_library.lvlib\\Stim_loaded"(w288) -> ()  [unwired: 1 in, 1 out]
      n271 = Subtract(x=w287, y=w291) -> (x-y=→"Lag1":dbl)
      n272 = shared-variable "My Computer\\michelle_library.lvlib\\InitiatedLag"(w287) -> ()  [unwired: 1 in, 1 out]
    }
  }
